vi "testInsertLastElement.vi"(8 "error in (no error)":errorcluster, 11 "TestCase in":refnum<class "ListImp_Common.lvclass">) -> (0 "error out":errorcluster, 3 "TestCase out":refnum<class "ListImp_Common.lvclass">)   [LabVIEW 2013, in "ListImp_Common.lvclass"]
uses:
  ListImp_Common.lvclass
  ListImp_Common.lvclass/ListImp_Common.ctl
  source/LapDog.Collections.Lists/ListImp/ListImp.lvclass
  <vilib>/addons/_JKI Toolkits/VI Tester/TestCase.llb/TestCase.lvclass
  source/LapDog.Collections.Common/I32/I32.lvclass
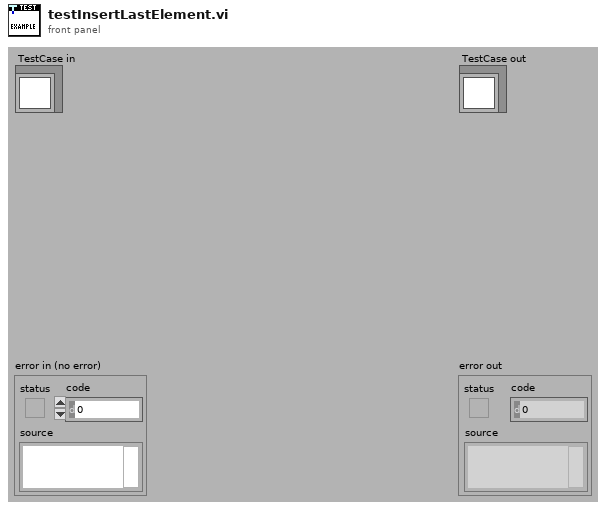
[diagram p1: front panel]
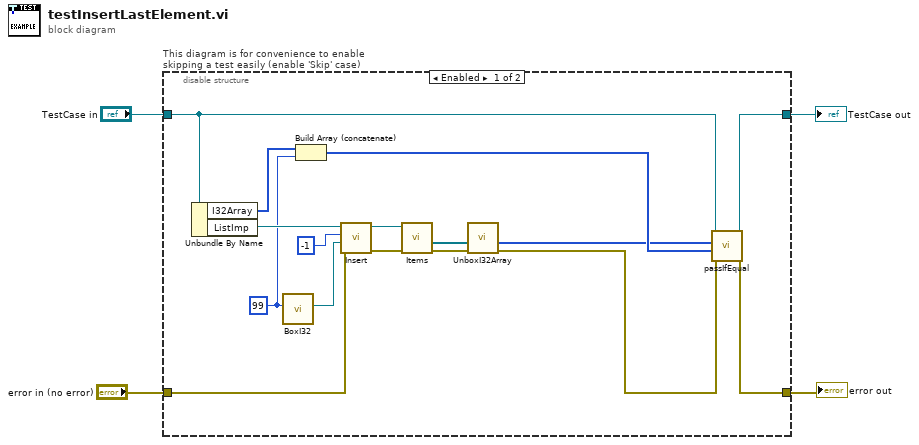
[diagram p0: block diagram]
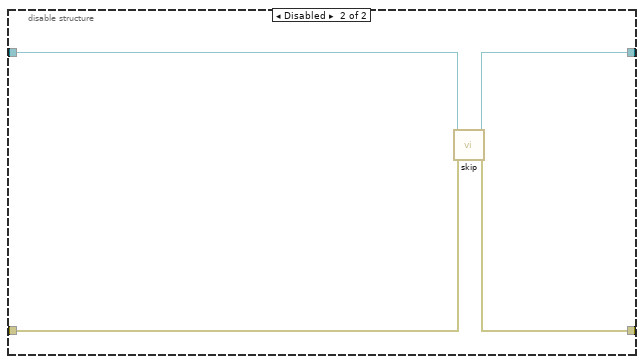
[diagram p2: hidden frame]
diagram:
  n1 = disable-structure "This diagram is for convenience to enable skipping a test easily (enable 'Skip' case)" shown="Enabled" {
    disable-tunnel: "TestCase in" -> [w18 w24]
    disable-tunnel: [w20 w22] -> w1
    disable-tunnel: [w19 w23] -> w3
    disable-tunnel: "error in (no error)" -> [w13 w21]
    frame Enabled {
      w10 = 99 ("Numeric")
      n2 = Unbundle By Name(w18) -> ("I32Array"=w11:i32[], "ListImp"=w17:refnum<class "ListImp.lvclass">)
      n3 = call "BoxI32.vi"("Numeric"=w10) -> ("I32 out"=w12:refnum<class "I32.lvclass">)  [unwired: 10 in]
      n4 = Build Array (concatenate)(w11, w10) -> (w9:i32[])
      n5 = call-dynamic "Insert.vi"("error in (no error)"=w13, "Item"=w12, "Index"=-1, "ListImp in"=w17) -> ("error out"=w14:errorcluster, "ListImp out"=w15:refnum<class "ListImp.lvclass">)  [unwired: 6 in]
      n6 = call-dynamic "Items.vi"("error in (no error)"=w14, "ListImp in"=w15) -> ("error out"=w8:errorcluster, "Items"=w6:refnum<class>[])  [unwired: 7 in, 1 out]
      n7 = call "UnboxI32Array.vi"("error in (no error)"=w8, "Items"=w6) -> ("error out"=w7:errorcluster, "Array"=w5:i32[])  [unwired: 8 in]
      n8 = call-dynamic "passIfEqual.vi"("error in (no error)"=w7, "y"=w9, "x"=w5, "TestCase in"=w18) -> ("error out"=w19:errorcluster, "TestCase out"=w20:refnum<class "ListImp_Common.lvclass">)  [unwired: 6 in]
    }
    frame Disabled {
      # "skip test result while test is under development"
      n9 = call <vilib>:"skip.vi"("error in (no error)"=w21, "TestCase in"=w24) -> ("error out"=w23:errorcluster, "TestCase out"=w22:refnum<class "ListImp_Common.lvclass">)  [unwired: 8 in]
    }
  }
  "error out" <- w3
  "TestCase out" <- w1
